vi "Main.vi"() -> ()   [LabVIEW 2021]
uses:
  Sudoku/Sudoku.lvclass/Sudoku.ctl
  Sudoku/Sudoku.lvclass
panel:
  out "display":picture
  in  "exit":bool
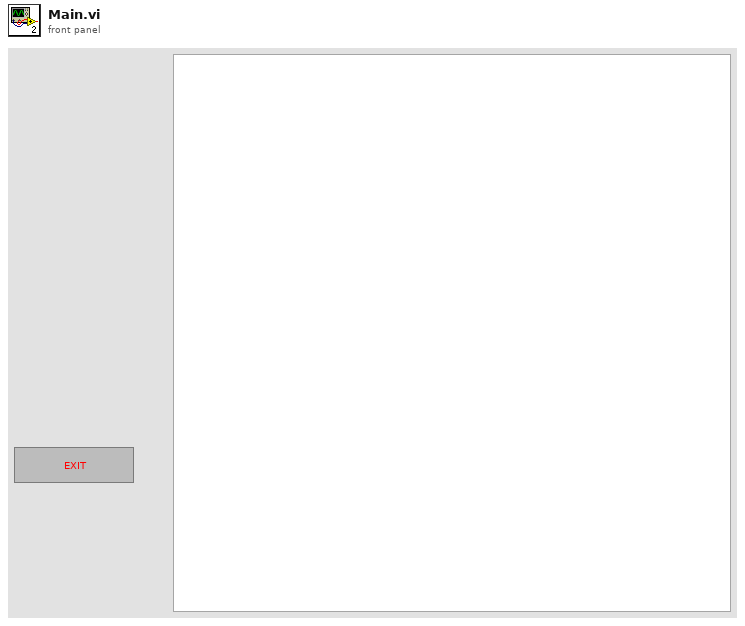
[diagram p1: front panel]
types:
  T1 = typedef "LVRectTypeDef.ctl" = cluster{"Left":i16, "Top":i16, "Right":i16, "Bottom":i16}
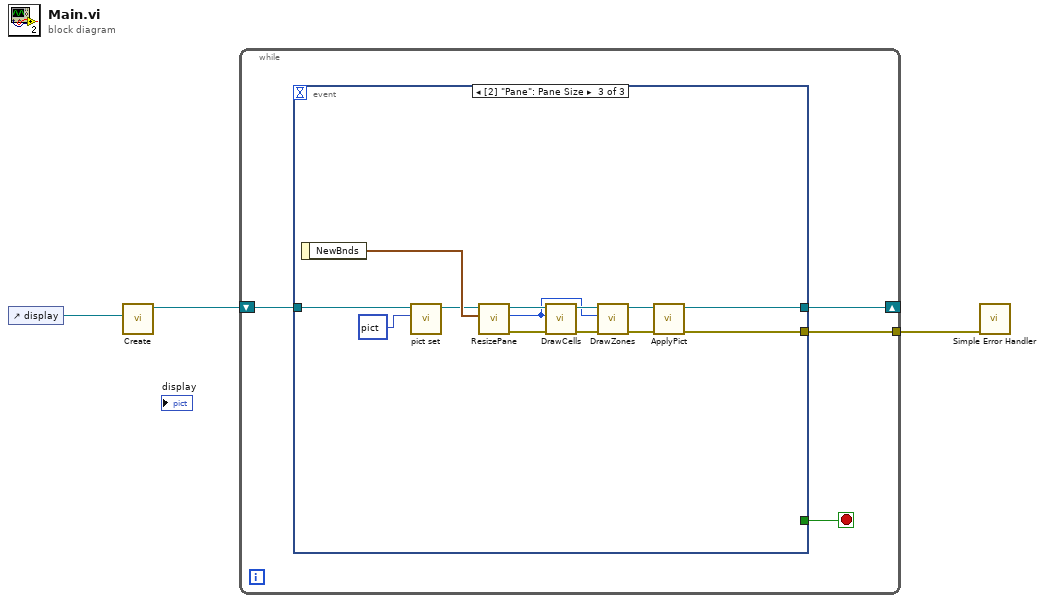
[diagram p0: block diagram]
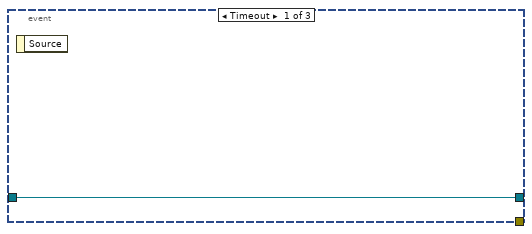
[diagram p2: hidden frame]
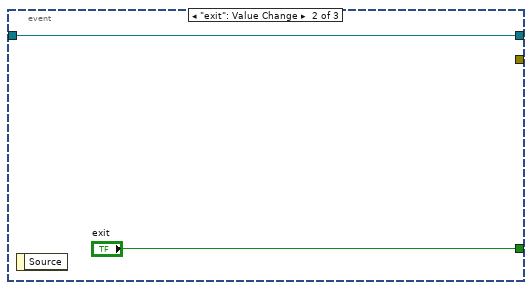
[diagram p3: hidden frame]
diagram:
  n1 = control-ref of="display"() -> (w3:refnum<vi>)
  n2 = call "Create.vi"("display ref"=w3) -> ("Sudoku.lvclass out"=w2:refnum<class "Sudoku.lvclass">)  [unwired: 10 in]
  n3 = while {
    shift-right: [w5] -> _
    shift-left: w2 -> [w6]
    tunnel: [w4] -> w1
    stop <- w7 stop-if-true
    n4 = event shown="[2] \"Pane\": Pane Size" {
      selector: _ -> [_ _ _]
      dyn-events: _ -> [_ _ _]
      timeout: _ -> [_ _ _]
      tunnel: [_ "exit" _] -> w7
      tunnel: w6 -> [w8 w9 w22]
      tunnel: [w8 w9 w17] -> w5
      tunnel: [_ _ w16] -> w4
      event Timeout {
        n5 = event-data() -> ()  [unwired: 1 in, 1 out]
      }
      event "exit": Value Change {
        n6 = event-data() -> ()  [unwired: 1 in, 1 out]
      }
      event Pane Size {
        n7 = event-data() -> ("NewBnds"=w23:T1)  [unwired: 1 in]
        n8 = call "pict set.vi"("picture"=picture data[5B], "Sudoku in"=w22) -> ("Sudoku out"=w21:refnum<class "Sudoku.lvclass">)  [unwired: 9 in]
        n9 = call "ResizePane.vi"("NewBnds"=w23, "Sudoku in"=w21) -> ("error out"=w19:errorcluster, "Cell Size"=w13:i32, "Sudoku out"=w20:refnum<class "Sudoku.lvclass">)  [unwired: 7 in]
        n10 = call "DrawCells.vi"("error in (no error)"=w19, "Cell Size"=w13, "Sudoku.lvclass in"=w20) -> ("error out"=w14:errorcluster, "Sudoku.lvclass out"=w15:refnum<class "Sudoku.lvclass">)  [unwired: 7 in]
        n11 = call "DrawZones.vi"("error in (no error)"=w14, "Cell Size"=w13, "Sudoku.lvclass"=w15) -> ("error out"=w12:errorcluster, "Sudoku.lvclass out"=w11:refnum<class "Sudoku.lvclass">)  [unwired: 7 in]
        n12 = call "ApplyPict.vi"("error in (no error)"=w12, "Sudoku in"=w11) -> ("error out"=w16:errorcluster, "Sudoku out"=w17:refnum<class "Sudoku.lvclass">)  [unwired: 8 in]
      }
    }
  }
  n13 = call <vilib>:"Simple Error Handler.vi"("error in (no error)"=w1) -> ()  [unwired: 4 in, 5 out]
